vi "stop_variable.vi"(8 "Error In":errorcluster, 9 "Write":bool, 11 "Enum":enum16{"read", "write"}(ring)) -> (0 "Error Out":errorcluster, 1 "read":bool)   [LabVIEW 2019]
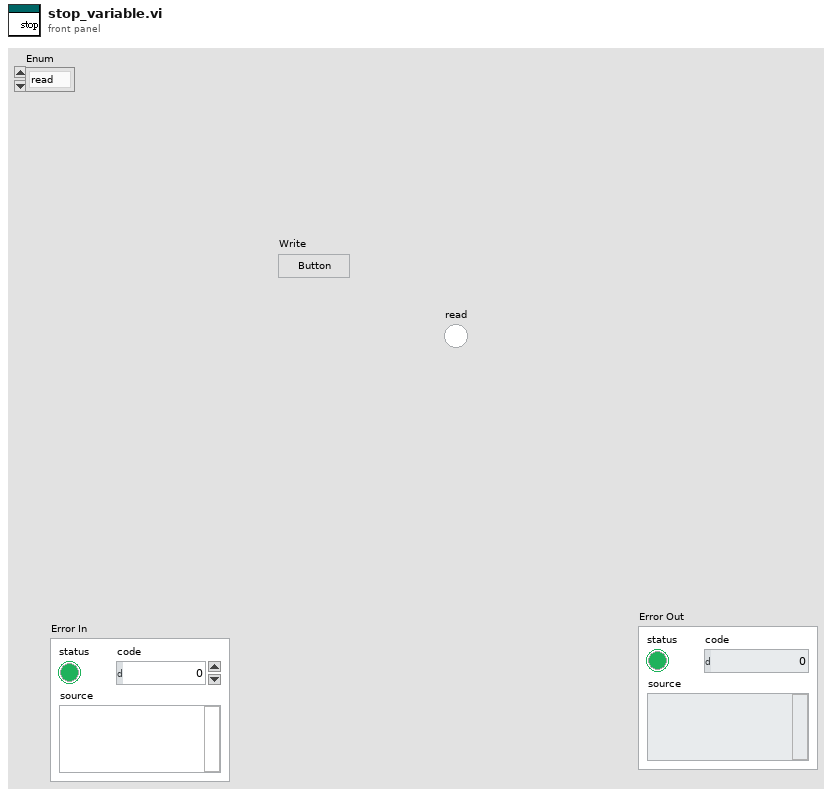
[diagram p1: front panel]
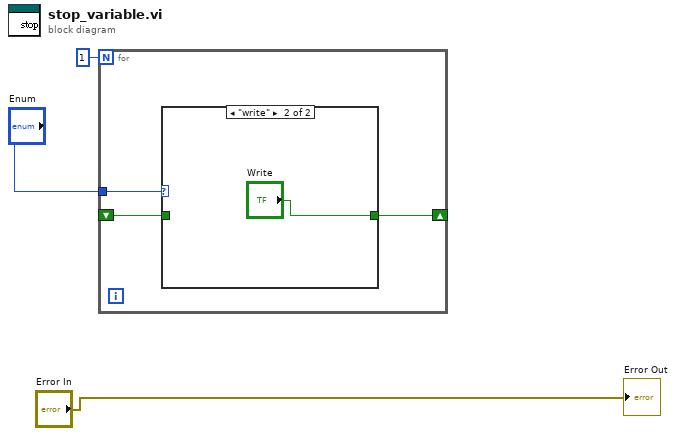
[diagram p0: block diagram]
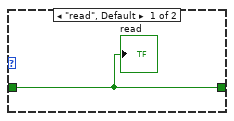
[diagram p2: hidden frame]
diagram:
  n1 = for {
    N: 1 -> [_]
    shift-right: [w5] -> _
    shift-left: _ -> [w4]
    tunnel: "Enum" -> [w6]
    n2 = case shown="\"write\"" w6 {
      tunnel: [w7 "Write"] -> w5
      tunnel: w4 -> [w7 _]
      frame "read", Default {
        "read" <- w7
      }
      frame "write" {
      }
    }
  }
  "Error Out" <- "Error In"
